vi "TracaHioki.vi"(8 "errin":errorcluster, 9 "datain":string, 10 "etage":string, 11 "PN":string) -> (0 "error out":errorcluster, 3 "out":string)   [LabVIEW 2020]
uses:
  VarGLO/Global var.vi
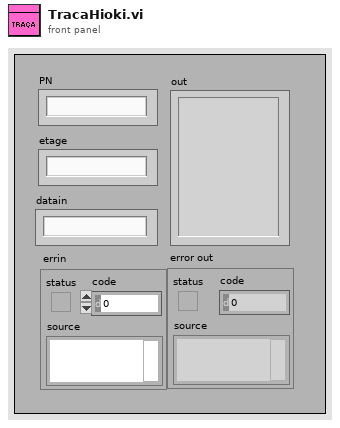
[diagram p1: front panel]
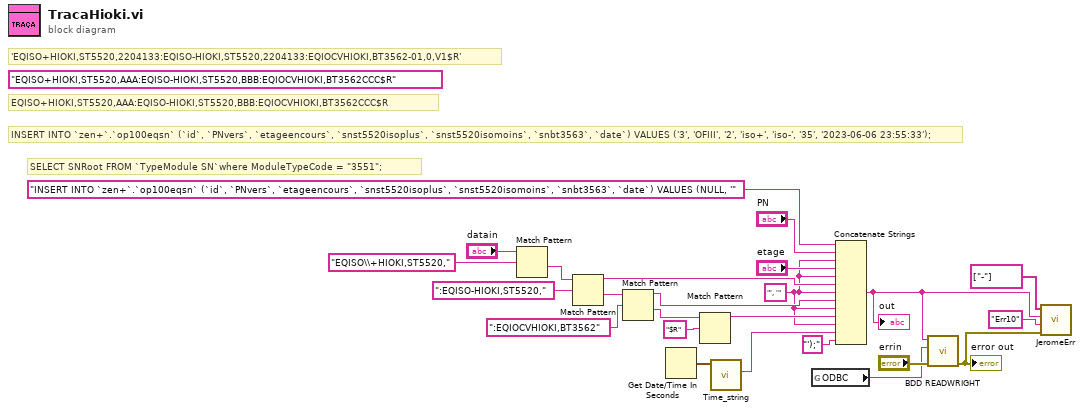
[diagram p0: block diagram]
diagram:
  w10 = "', '" ("chaîne")
  (unwired) "EQISO+HIOKI,ST5520,AAA:EQISO-HIOKI,ST5520,BBB:EQIOCVHIOKI,BT3562CCC$R" ("chaîne")
  # "'EQISO+HIOKI,ST5520,2204133:EQISO-HIOKI,ST5520,2204133:EQIOCVHIOKI,BT3562-01,0,V1$R'"
  # "EQISO+HIOKI,ST5520,AAA:EQISO-HIOKI,ST5520,BBB:EQIOCVHIOKI,BT3562CCC$R"
  # "INSERT INTO `zen+`.`op100eqsn` (`id`, `PNvers`, `etageencours`, `snst5520isoplus`, `snst5520isomoins`, `snbt3563`, `date`) VALUES ('3', 'OFIII', '2', 'iso+', 'iso-', '35', '2023-06-06 23:55:33');"
  # "SELECT SNRoot FROM `TypeModule SN`where ModuleTypeCode = \"3551\";"
  n1 = Match Pattern ("Rechercher une expression")(string="datain", regular expression="EQISO\\+HIOKI,ST5520," ("expression régulière")) -> (after substring=w16:string)  [unwired: 1 in, 3 out]
  n2 = Match Pattern ("Rechercher une expression")(string=w16, regular expression=":EQISO-HIOKI,ST5520," ("expression régulière")) -> (before substring=w13:string, after substring=w22:string)  [unwired: 1 in, 2 out]
  n3 = Match Pattern ("Rechercher une expression")(string=w22, regular expression=":EQIOCVHIOKI,BT3562" ("expression régulière")) -> (before substring=w12:string, after substring=w20:string)  [unwired: 1 in, 2 out]
  n4 = Get Date/Time In Seconds() -> (seconds since 1Jan1904=w9:timestamp)
  n5 = Match Pattern ("Rechercher une expression")(string=w20, regular expression="$R" ("expression régulière")) -> (before substring=w11:string)  [unwired: 1 in, 3 out]
  n6 = call <vilib>:"Time_string.vi"("h in"=w9) -> ("heure sql"=w8:string)  [unwired: 9 in, 1 out]
  n7 = global read "Global var.vi" "ODBC"() -> (w1:string)
  n8 = Concatenate Strings("INSERT INTO `zen+`.`op100eqsn` (`id`, `PNvers`, `etageencours`, `snst5520isoplus`, `snst5520isomoins`, `snbt3563`, `date`) VALUES (NULL, '" ("SQL query"), "PN", w10, "etage", w10, w13, w10, w12, w10, w11, w10, w8, "');" ("chaîne")) -> (w3:string)
  "out" <- w3
  n9 = call <userlib>:"BDD READWRIGHT.vi"("errin"="errin", "DSN name"=w1, "Instruction"=w3) -> ("error out"=w2:errorcluster)  [unwired: 7 in, 1 out]
  "error out" <- w2
  n10 = call "JeromeErr.vi"("Errin"=w2, "CodeERR"="Err10", "RequetteSQL"=w3, "RetourSQL"=string[] ["-"]) -> ()  [unwired: 8 in]
